vi "Delete SBlock.vi"(8 "error in (no error)":errorcluster, 10 "index":i32, 11 "Sequence of SBlocks in":refnum<class "Sequence of SBlocks.lvclass">) -> (0 "error out":errorcluster, 2 "Schedule Block":refnum<class "Schedule Block.lvclass">, 3 "Sequence of SBlocks out":refnum<class "Sequence of SBlocks.lvclass">)   [LabVIEW 2020, in "TALOS.lvlib" / "Run Utilities.lvlib" / "Sequence of SBlocks.lvclass"]
uses:
  Sequence of SBlocks.lvclass
  Schedule Block/Schedule Block.lvclass
  Sequence of SBlocks.lvclass/Sequence of SBlocks.ctl
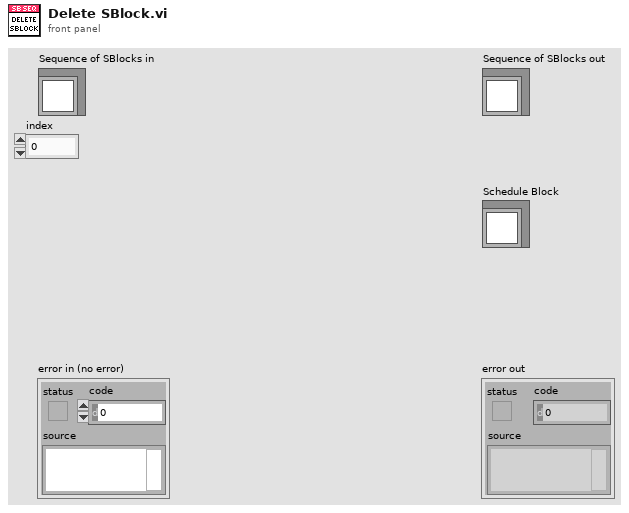
[diagram p1: front panel]
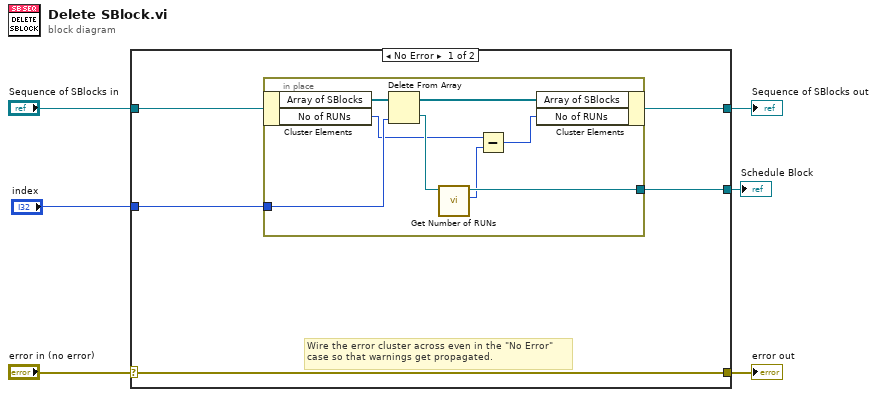
[diagram p0: block diagram]
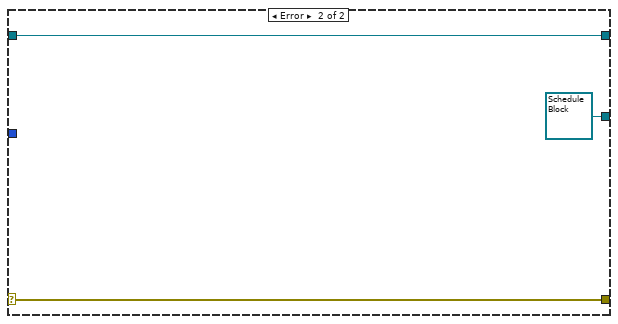
[diagram p2: hidden frame]
diagram:
  n1 = case shown="No Error" "error in (no error)" {
    selector: "error in (no error)" -> [w11 w22]
    tunnel: [w11 w22] -> w5
    tunnel: [w9 w21] -> w3
    tunnel: "Sequence of SBlocks in" -> [w10 w21]
    tunnel: "index" -> [w8 _]
    tunnel: [w7 refnum<class "Schedule Block.lvclass"> refnum ("Run Utilities.lvlib:Schedule Block.lvclass")] -> w1
    frame No Error {
      # "Wire the error cluster across even in the \"No Error\"\ncase so that warnings get propagated."
      n2 = in-place {
        in-place-border: w8 -> [w17]
        in-place-border: [w15] -> w7
        n3 = in-place-cluster #1(w10) -> ("Array of SBlocks"=w19:refnum<class "Schedule Block.lvclass">[], "No of RUNs"=w14:i32)
        n4 = Delete From Array(array=w19, index=w17) -> (deleted portion=w16:refnum<class "Schedule Block.lvclass">, array with subset deleted=w18:refnum<class "Schedule Block.lvclass">[])  [unwired: 1 in]
        n5 = call-dynamic "Get Number of RUNs.vi"("Schedule Block in"=w16) -> ("No. of RUNs"=w13:i32, "Schedule Block out"=w15:refnum<class "Schedule Block.lvclass">)  [unwired: 8 in, 1 out]
        n6 = Subtract(x=w14, y=w13) -> (x-y=w12:i32)
        n7 = in-place-cluster #1("Array of SBlocks"=w18, "No of RUNs"=w12) -> (w9:refnum<class "Sequence of SBlocks.lvclass">)
      }
    }
    frame Error {
    }
  }
  "error out" <- w5
  "Sequence of SBlocks out" <- w3
  "Schedule Block" <- w1
